vi "Main.vi"   [LabVIEW 2020]
doc: "This simulates the functionality of an ATM cash dispenser."
uses:
  GUI/GUI.lvlib
  Hardware/Hardware.lvlib
  Manager/Manager.lvlib
panel:
  # "Module MAIN VI (Launcher)"
types:
  T1 = enum32{"Invalid", "Standard", "Closed", "Hidden", "Minimized", "Maximized"}
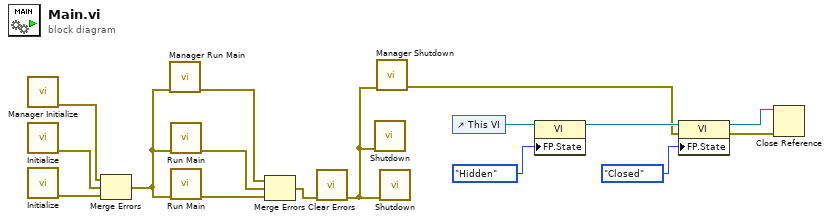
[diagram p0: block diagram]
diagram:
  n1 = call "Manager Initialize.vi"() -> ("error out"=w6:errorcluster)  [unwired: 11 in]
  n2 = call "Initialize.vi"() -> ("error out"=w16:errorcluster)  [unwired: 11 in]
  n3 = call "Initialize.vi"() -> ("error out"=w1:errorcluster)  [unwired: 11 in]
  n4 = Merge Errors(w6, w16, w1) -> (w5:errorcluster)
  n5 = call "Manager Run Main.vi"("error in"=w5) -> ("error out"=w4:errorcluster)  [unwired: 10 in]
  n6 = call "Run Main.vi"("error in"=w5) -> ("error out"=w15:errorcluster)  [unwired: 10 in]
  n7 = call "Run Main.vi"("error in"=w5) -> ("error out"=w7:errorcluster)  [unwired: 10 in]
  n8 = Merge Errors(w4, w15, w7) -> (w8:errorcluster)
  n9 = call <vilib>:"Clear Errors.vi"("error in (no error)"=w8) -> ("error out"=w3:errorcluster)  [unwired: 5 in, 1 out]
  n10 = call "Shutdown.vi"("error in"=w3) -> ()  [unwired: 10 in, 1 out]
  n11 = call "Manager Shutdown.vi"("error in"=w3) -> ("error out"=w2:errorcluster)  [unwired: 10 in]
  n12 = call "Shutdown.vi"("error in"=w3) -> ()  [unwired: 10 in, 1 out]
  n13 = control-ref of="This VI"() -> (w14:refnum<vi>)
  n14 = property on="Property Node" class="VI"(reference=w14, "FP.State"=T1."Hidden" ("Front Panel Window:State")) -> (reference out=w11:refnum<vi>)  [unwired: 1 in, 1 out]
  n15 = property on="Property Node" class="VI"(reference=w11, error in=w2, "FP.State"=T1."Closed" ("Front Panel Window:State")) -> (reference out=w10:refnum<vi>, error out=w12:errorcluster)
  n16 = Close Reference(reference=w10, error in (no error)=w12) -> ()  [unwired: 1 out]
